vi "ListenToCD.vi"(8 "error in (no error)":errorcluster, 11 "Facade in":refnum<class "Facade.lvclass">) -> (0 "error out":errorcluster, 2 "ProcessMessage":string, 3 "Facade out":refnum<class "Facade.lvclass">)   [LabVIEW 2013, in "Facade.lvclass"]
uses:
  Facade.lvclass
  Facade.lvclass/Facade.ctl
  RoomLight.lvclass/RoomLight.lvclass
  Tuner.lvclass/Tuner.lvclass
  DVDPlayer.lvclass/DVDPlayer.lvclass
  Projector.lvclass/Projector.lvclass
  CDPlayer.lvclass/CDPlayer.lvclass
  Amplifer.lvclass/Amplifer.lvclass
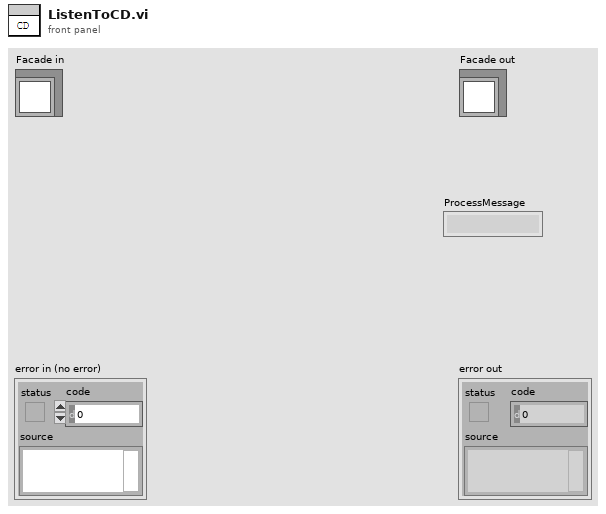
[diagram p1: front panel]
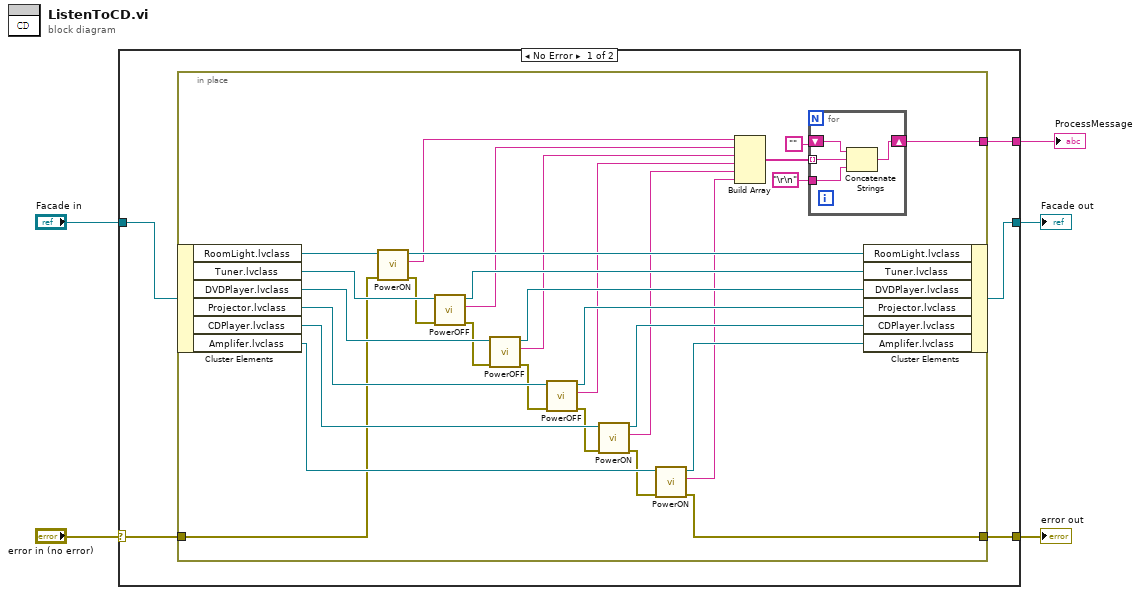
[diagram p0: block diagram]
diagram:
  n1 = case shown="No Error" "error in (no error)" {
    selector: "error in (no error)" -> [w10 w45]
    tunnel: [w6 w45] -> w4
    tunnel: [w8 w44] -> w2
    tunnel: "Facade in" -> [w9 w44]
    tunnel: [w7 _] -> w1
    frame No Error {
      n2 = in-place {
        in-place-border: w10 -> [w29]
        in-place-border: [w36] -> w7
        in-place-border: [w11] -> w6
        n3 = in-place-cluster #1(w9) -> ("RoomLight.lvclass"=w35:refnum<class "RoomLight.lvclass">, "Tuner.lvclass"=w34:refnum<class "Tuner.lvclass">, "DVDPlayer.lvclass"=w33:refnum<class "DVDPlayer.lvclass">, "Projector.lvclass"=w32:refnum<class "Projector.lvclass">, "CDPlayer.lvclass"=w31:refnum<class "CDPlayer.lvclass">, "Amplifer.lvclass"=w30:refnum<class "Amplifer.lvclass">)
        n4 = call-dynamic "PowerON.vi"("error in (no error)"=w29, "RoomLight in"=w35) -> ("error out"=w28:errorcluster, "Message"=w12:string, "RoomLight out"=w23:refnum<class "RoomLight.lvclass">)  [unwired: 7 in]
        n5 = call-dynamic "PowerOFF.vi"("error in (no error)"=w28, "Tuner in"=w34) -> ("error out"=w27:errorcluster, "Message"=w13:string, "Tuner out"=w22:refnum<class "Tuner.lvclass">)  [unwired: 7 in]
        n6 = call-dynamic "PowerOFF.vi"("error in (no error)"=w27, "DVDPlayer in"=w33) -> ("error out"=w26:errorcluster, "Message"=w14:string, "DVDPlayer out"=w21:refnum<class "DVDPlayer.lvclass">)  [unwired: 7 in]
        n7 = call-dynamic "PowerOFF.vi"("error in (no error)"=w26, "Projector in"=w32) -> ("error out"=w25:errorcluster, "Message"=w15:string, "Projector out"=w20:refnum<class "Projector.lvclass">)  [unwired: 7 in]
        n8 = call-dynamic "PowerON.vi"("error in (no error)"=w25, "CDPlayer in"=w31) -> ("error out"=w24:errorcluster, "Message"=w16:string, "CDPlayer out"=w19:refnum<class "CDPlayer.lvclass">)  [unwired: 7 in]
        n9 = call-dynamic "PowerON.vi"("error in (no error)"=w24, "Amplifer in"=w30) -> ("error out"=w11:errorcluster, "Message"=w17:string, "Amplifer out"=w18:refnum<class "Amplifer.lvclass">)  [unwired: 7 in]
        n10 = Build Array(w12, w13, w14, w15, w16, w17) -> (w39:string[])
        n11 = for {
          tunnel: w39 -> [w40] mode=indexing
          tunnel: "\r\n" -> [w43]
          shift-right: [w41] -> w36
          shift-left: "" -> [w42]
          n12 = Concatenate Strings(w42, w40, w43) -> (w41:string)
        }
        n13 = in-place-cluster #1("RoomLight.lvclass"=w23, "Tuner.lvclass"=w22, "DVDPlayer.lvclass"=w21, "Projector.lvclass"=w20, "CDPlayer.lvclass"=w19, "Amplifer.lvclass"=w18) -> (w8:refnum<class "Facade.lvclass">)
      }
    }
    frame Error {
    }
  }
  "error out" <- w4
  "Facade out" <- w2
  "ProcessMessage" <- w1
